vi "svc_Engineering Units to Unit Label.vi"(10 "custom label":string="EU", 11 "engineering units":T2=1 items=["custom..."=0, "V"=1, "A"=21, "C"=30, "pC"=31, "s"=32, "-"=29, "Pa"=2, "N"=20, "g"=3, "m/s^2"=4, "m/s"=5, "m"=6, "mm/s"=12, "mm"=13, "micron/s"=14, "micron"=15, "in/s^2"=7, "in/s"=8, "in"=9, "mil/s"=10, "mil"=11, "rad/s^2"=16, "rad/s"=17, "rad"=18, "deg/s^2"=26, "deg/s"=27, "deg"=28, "RPM"=22, "cycle/s^2"=23, "Hz"=24, "cycle"=25, "strain"=19]) -> (2 "unit label":string="EU", 3 "engineering units enum":T1(ring)=enum."V")   [LabVIEW 2017]
uses:
  <vilib>/addons/_NISVFA/_Shared subVIs/Controls/svc_Engineering Units Text Ring.ctl
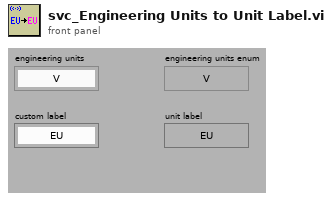
[diagram p1: front panel]
types:
  T1 = enum16{"custom...", "V", "Pa", "g", "m/s^2", "m/s", "m", "in/s^2", "in/s", "in", "mil/s", "mil", "mm/s", "mm", "micron/s", "micron", "rad/s^2", "rad/s", "rad", "strain", "N", "A", "rpm", "cycle/s^2", "Hz", "cycle", "deg/s^2", "deg/s", "deg", "Undefined", "C", "pC"}
  T2 = typedef "svc_Engineering Units Text Ring.ctl" = u16
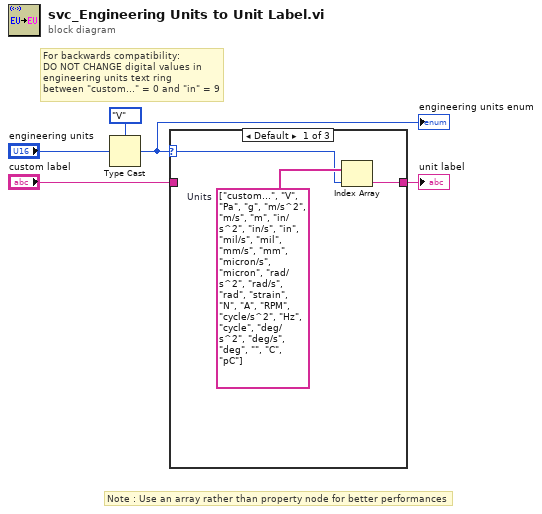
[diagram p0: block diagram]
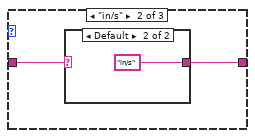
[diagram p2: hidden frame]
diagram:
  # "For backwards compatibility:\nDO NOT CHANGE digital values in \nengineering units text ring\nbetween \"custom...\" = 0 and \"in\" = 9"
  # "Note : Use an array rather than property node for better performances"
  n1 = Type Cast(type=T1."V" ("engineering units enum"), x="engineering units") -> (*(type *) &x=w2:T1)
  "engineering units enum" <- w2
  n2 = case shown="Default" w2 {
    selector: w2 -> [w6 _ _]
    tunnel: [w7 w9 w13] -> w4
    tunnel: "custom label" -> [_ w10 w13]
    frame Default {
      w8 = string[] ["custom...", "V", "Pa", "g", "m/s^2", "m/s", "m", "in/s^2", "in/s", "in", "mil/s", "mil", "mm/s", "mm", "micron/s", "micron", "rad/s^2", "rad/s", "rad", "strain", "N", "A", "RPM", "cycle/s^2", "Hz", "cycle", "deg/s^2", "deg/s", "deg", "", "C", "pC"]  # Units
      n3 = Index Array(array=w8, index=w6) -> (element=w7:string)
    }
    frame "in/s" {
      n4 = case shown="Default" w10 {
        selector: w10 -> [w11 _]
        tunnel: [w11 "in/s" ("t")] -> w9
        frame "ips" {
        }
        frame Default {
        }
      }
    }
    frame "custom..." {
    }
  }
  "unit label" <- w4
